vi "_26_Sample_qsns_9[2].vi"() -> ()   [LabVIEW 2020]
panel:
  in  "stop":bool
  out "x":i32
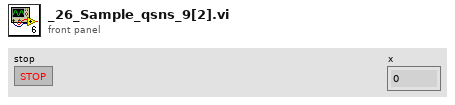
[diagram p1: front panel]
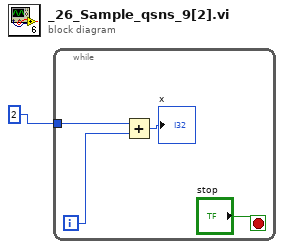
[diagram p0: block diagram]
diagram:
  n1 = while {
    tunnel: 2 -> [w5]
    i -> [w4]
    stop <- "stop" stop-if-true
    n2 = Add(x=w5, y=w4) -> (x+y=→"x":i32)
  }
